vi "HAL camera get one frame - SubVI.vi"(2 "error in":errorcluster, 3 "New Image":T1, 4 "Camera Parameters (important)":T2={"Exposure Time (sec)"=0.0, "EM CCD Gain"=0, "Readout Settings"={"Acquisition Mode"=enum."(do not use)", "Pixel Rate"=enum."EM CCD 10 Mhz 14 bits", "High Capacity?"=FALSE, "V Shift Speed (us/row)"=enum."0.9 (not reccommended)", "V Shift Amplitude"=enum."normal", "Preamp Gain"=enum."2.4", "Trigger Mode"=0}, "Image Size"={"H Bin"=0, "V Bin"=0, "Left"=0, "Top"=0, "Right"=0, "Bottom"=0}, "Shutter"=0} {"Shutter" items=["Auto", "Stay Open", "Always Closed"]; "Readout Settings"."Trigger Mode" items=["Internal", "External"]; "EM CCD Gain" scale=1.0..300.0; "Exposure Time (sec)" scale=0.001..10.0 scale format="%#_1g"}) -> (0 "error out":errorcluster, 1 "Image Out":T1)   [LabVIEW 2014]
uses:
  Glimpse-master/Microscope plugins/ixon1024/HAL camera parameters important.ctt
  <vilib>/vision/Image Controls.llb/IMAQ Image.ctl
  Glimpse-master/Microscope plugins/ixon1024/andor acquisition mode.ctl
  Glimpse-master/Microscope plugins/ixon1024/ixon readout settings.ctl
panel:
  # "Camera: Andor iXon"
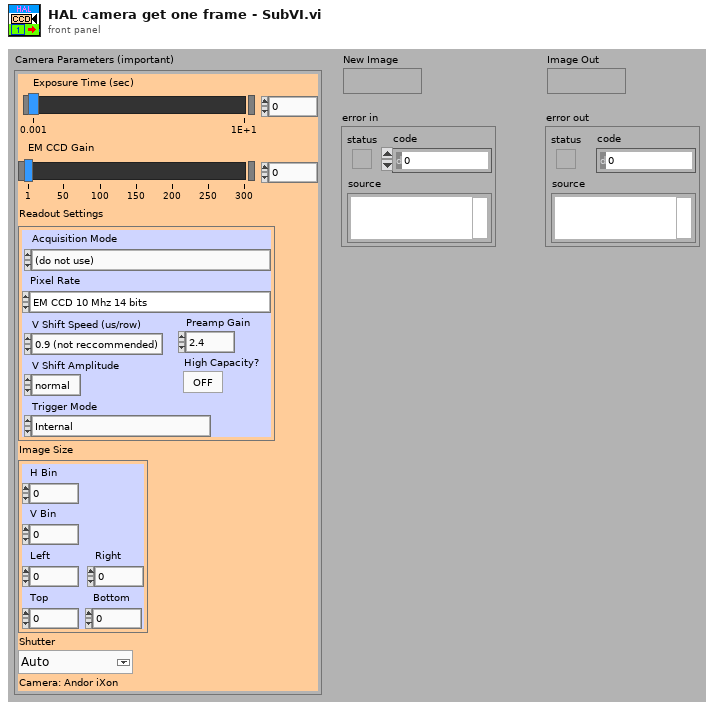
[diagram p1: front panel]
types:
  T1 = typedef "IMAQ Image.ctl" = refnum<image>
  T2 = typedef "HAL camera parameters important.ctt" = cluster{"Exposure Time (sec)":sgl, "EM CCD Gain":u16, "Readout Settings":T3, "Image Size":cluster{"H Bin":i32, "V Bin":i32, "Left":i32, "Top":i32, "Right":i32, "Bottom":i32}, "Shutter":i32}
  T3 = typedef "ixon readout settings.ctl" = cluster{"Acquisition Mode":T4, "Pixel Rate":enum16{"EM CCD 10 Mhz 14 bits", "EM CCD 5 Mhz 14 bits", "EM CCD 3 Mhz 14 bits", "EM CCD 1 Mhz 16 bits", "Standard CCD 3 Mhz 14 bits", "Standard CCD 1 Mhz 16 bits"}, "High Capacity?":bool, "V Shift Speed (us/row)":enum16{"0.9 (not reccommended)", "1.7  (not reccommended)", "3.3  (not reccommended)", "6.5", "12.9"}, "V Shift Amplitude":enum16{"normal", "+1", "+2", "+3", "+4"}, "Preamp Gain":enum16{"1.0", "2.4", "5.0"}, "Trigger Mode":u32}
  T4 = typedef "andor acquisition mode.ctl" = enum16{"(do not use)", "Single Scan", "Accumulate", "Kinetics", "Fast Kinetics", "Kinetics Run till Abort", "Frame Transfer", "Frame Transfer Run till Abort", "(do not use) ", "Time Delayed Integration"}
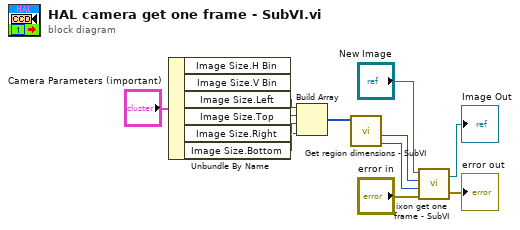
[diagram p0: block diagram]
diagram:
  n1 = Unbundle By Name("Camera Parameters (important)") -> ("Image Size.Left"=w10:i32, "Image Size.Top"=w9:i32, "Image Size.Right"=w8:i32, "Image Size.Bottom"=w7:i32)  [unwired: 2 out]
  n2 = Build Array(w10, w9, w8, w7) -> (w11:i32[])
  n3 = call "Get region dimensions - SubVI.vi"("x1y1x2y2"=w11) -> ("y size"=w2:u16, "x size"=w3:u16)  [unwired: 7 in, 2 out]
  n4 = call "ixon get one frame - SubVI.vi"("error in"="error in", "Image Height"=w2, "Image Width"=w3, "Image In"="New Image") -> ("error out"=→"error out":errorcluster, "Image Out"=→"Image Out":T1)  [unwired: 2 in]
